vi "Build DAQmx Lines.vi"(6 "Line (Range End)":i32, 7 "Line (Single - Range Start)":i32, 8 "error in (no error)":errorcluster, 9 "DAQmx Digital Scope":T1, 10 "DAQmx Lines Scope":T2, 11 "PXI6521 in":refnum<class "PXI6521.lvclass">) -> (0 "error out":errorcluster, 2 "Full Line":string, 3 "PXI6521 out":refnum<class "PXI6521.lvclass">)   [LabVIEW 2018, in "PXI6521.lvlib" / "PXI6521.lvclass"]
uses:
  PXI6521.lvclass
  Custom Controls/DAQmx Lines Scope.ctl
  Custom Controls/DAQmx Digital Scope.ctl
  PPLs/DigitalIO/Parent/DigitalIO.lvlibp/DigitalIO.lvclass
  PPLs/DigitalIO/Parent/Configuration.lvlibp/Configuration.lvclass
  C:/Projects/LabVIEW/PPLs/DigitalIO/Parent/DigitalIO.lvlibp/DigitalIO.lvclass
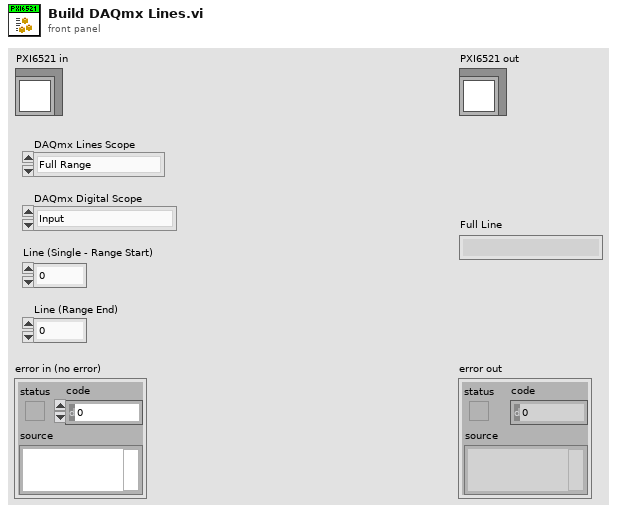
[diagram p1: front panel]
types:
  T1 = typedef "PXI6521.lvlib/PXI6521.lvclass/DAQmx Digital Scope.ctl" = enum16{"Input", "Output"}
  T2 = typedef "PXI6521.lvlib/PXI6521.lvclass/DAQmx Lines Scope.ctl" = enum16{"Full Range", "Custom Range", "Single"}
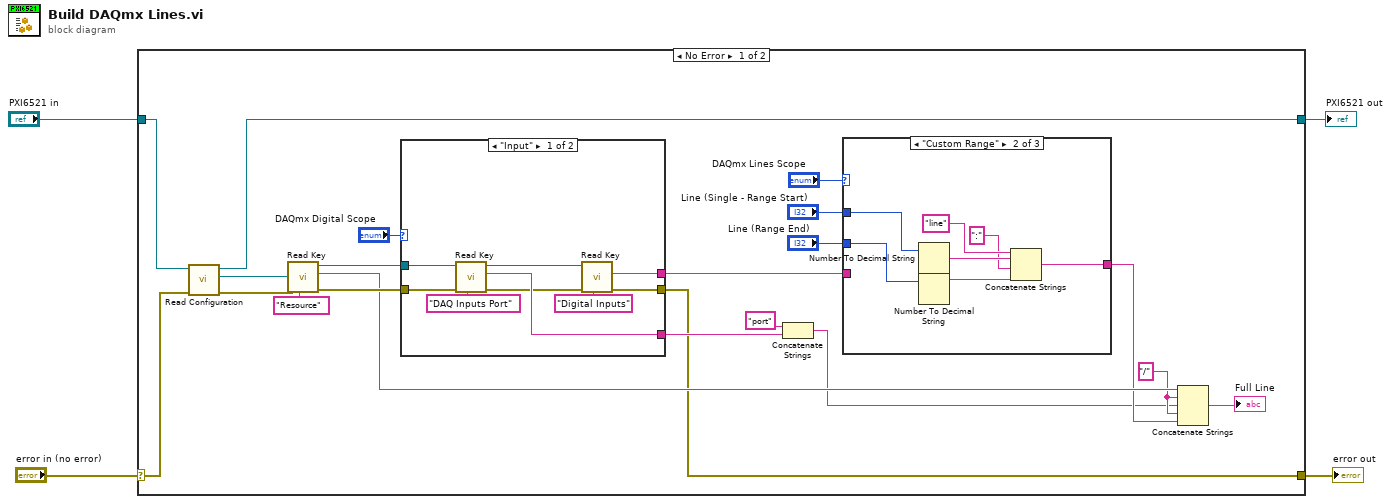
[diagram p0: block diagram]
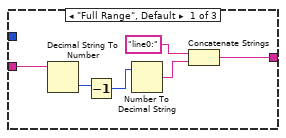
[diagram p2: hidden frame]
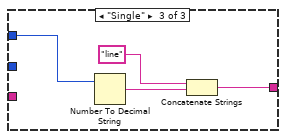
[diagram p3: hidden frame]
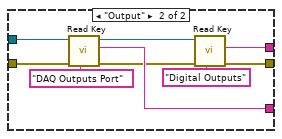
[diagram p4: hidden frame]
diagram:
  n1 = case shown="No Error" "error in (no error)" {
    selector: "error in (no error)" -> [w23 w62]
    tunnel: [w6 w62] -> w3
    tunnel: [w5 w61] -> w1
    tunnel: "PXI6521 in" -> [w22 w61]
    frame No Error {
      w14 = "/"
      n2 = call "Read Configuration.vi"("error in (no error)"=w23, "DigitalIO in"=w22) -> ("error out"=w8:errorcluster, "Configuration"=w7:refnum<class "Configuration.lvclass">, "DigitalIO out"=w5:refnum<class "PXI6521.lvclass">)  [unwired: 7 in]
      n3 = call "Read Key.vi"("Key:"="Resource", "error in"=w8, "Configuration in"=w7) -> ("error out"=w24:errorcluster, "Value"=w16:string, "Configuration out"=w25:refnum<class "Configuration.lvclass">)  [unwired: 6 in]
      n4 = case shown="\"Input\"" "DAQmx Digital Scope" {
        tunnel: w25 -> [w51 w60]
        tunnel: w24 -> [w50 w59]
        tunnel: [w49 w58] -> w12
        tunnel: [w48 w57] -> w6
        tunnel: [w47 w56] -> w19
        frame "Input" {
          n5 = call "Read Key.vi"("Key:"="DAQ Inputs Port", "error in"=w50, "Configuration in"=w51) -> ("error out"=w44:errorcluster, "Value"=w49:string, "Configuration out"=w43:refnum<class "Configuration.lvclass">)  [unwired: 6 in]
          n6 = call "Read Key.vi"("Key:"="Digital Inputs", "error in"=w44, "Configuration in"=w43) -> ("error out"=w48:errorcluster, "Value"=w47:string)  [unwired: 6 in, 1 out]
        }
        frame "Output" {
          n7 = call "Read Key.vi"("Key:"="DAQ Outputs Port", "error in"=w59, "Configuration in"=w60) -> ("error out"=w53:errorcluster, "Value"=w58:string, "Configuration out"=w52:refnum<class "Configuration.lvclass">)  [unwired: 6 in]
          n8 = call "Read Key.vi"("Key:"="Digital Outputs", "error in"=w53, "Configuration in"=w52) -> ("error out"=w57:errorcluster, "Value"=w56:string)  [unwired: 6 in, 1 out]
        }
      }
      n9 = Concatenate Strings("port" ("string"), w12) -> (w11:string)
      n10 = case shown="\"Custom Range\"" "DAQmx Lines Scope" {
        tunnel: w19 -> [w31 _ _]
        tunnel: [w26 w32 w39] -> w15
        tunnel: "Line (Single - Range Start)" -> [_ w37 w42]
        tunnel: "Line (Range End)" -> [_ w38 _]
        frame "Full Range", Default {
          n11 = Decimal String To Number(string=w31) -> (number=w30:i32)  [unwired: 2 in, 1 out]
          n12 = Decrement(x=w30) -> (x-1=w29:i32)
          n13 = Number To Decimal String(number=w29) -> (decimal integer string=w27:string)  [unwired: 1 in]
          n14 = Concatenate Strings("line0:", w27) -> (w26:string)
        }
        frame "Custom Range" {
          n15 = Number To Decimal String(number=w37) -> (decimal integer string=w35:string)  [unwired: 1 in]
          n16 = Number To Decimal String(number=w38) -> (decimal integer string=w33:string)  [unwired: 1 in]
          n17 = Concatenate Strings("line", w35, ":", w33) -> (w32:string)
        }
        frame "Single" {
          n18 = Number To Decimal String(number=w42) -> (decimal integer string=w40:string)  [unwired: 1 in]
          n19 = Concatenate Strings("line", w40) -> (w39:string)
        }
      }
      n20 = Concatenate Strings(w16, w14, w11, w14, w15) -> (→"Full Line":string)
    }
    frame Error {
    }
  }
  "error out" <- w3
  "PXI6521 out" <- w1
